vi "set phase sampling info duty cycle.vi"(8 "error in (no error)":errorcluster, 11 "Waveform in":refnum<class "Waveform.lvclass">) -> (0 "error out":errorcluster, 3 "Waveform out":refnum<class "Waveform.lvclass">)   [LabVIEW 2012, in "Waveform.lvclass"]
uses:
  Waveform.lvclass
  Waveform.lvclass/Waveform.ctl
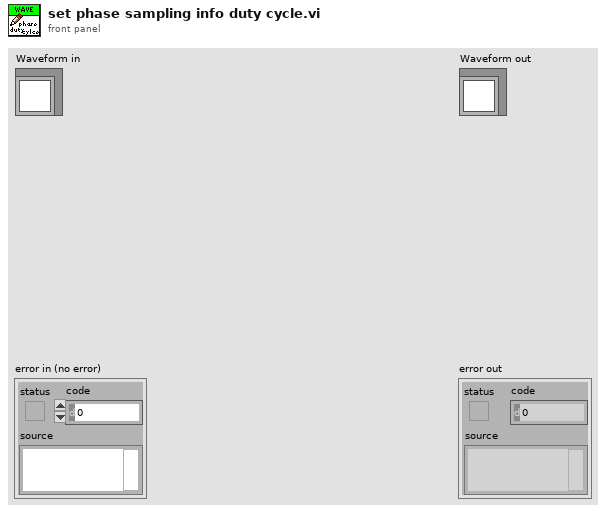
[diagram p1: front panel]
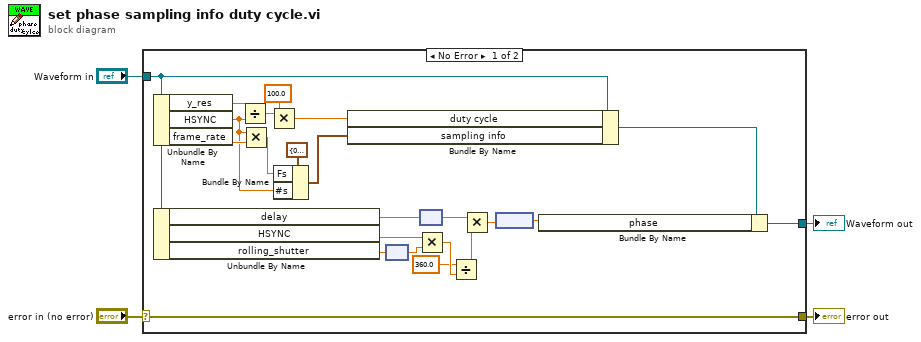
[diagram p0: block diagram]
diagram:
  n1 = case shown="No Error" "error in (no error)" {
    selector: "error in (no error)" -> [w27 w29]
    tunnel: [w27 w29] -> w3
    tunnel: [w11 w28] -> w1
    tunnel: "Waveform in" -> [w17 w28]
    frame No Error {
      n2 = Unbundle By Name(w17) -> ("y_res"=w26:dbl, "HSYNC"=w19:dbl, "frame_rate"=w22:dbl)
      n3 = Unbundle By Name(w17) -> ("delay"=w16:dbl[unit], "HSYNC"=w8:dbl, "rolling_shutter"=w10:dbl[unit])
      n4 = Divide(x=w26, y=w19) -> (x/y=w25:dbl)
      n5 = Multiply(x=w19, y=w22) -> (x*y=w20:dbl)
      n6 = Multiply(x=w25, y=100.0) -> (x*y=w23:dbl)
      n7 = Bundle By Name(cluster=cluster{"Fs":dbl, "#s":dbl} {"Fs"=0.0, "#s"=0.0} ("settings.Pockels Cell.sampling info"), "Fs"=w20, "#s"=w19) -> (w18:cluster{"Fs":dbl, "#s":dbl})
      n8 = Bundle By Name(cluster=w17, "duty cycle"=w23, "sampling info"=w18) -> (w12:refnum<class "Waveform.lvclass">)
      n9 = node(w10) -> (w9:dbl)
      n10 = Multiply(x=w8, y=w9) -> (x*y=w7:dbl)
      n11 = node(w16) -> (w15:dbl)
      n12 = Divide(x=360.0, y=w7) -> (x/y=w5:dbl)
      n13 = Multiply(x=w15, y=w5) -> (x*y=w14:dbl)
      n14 = node(w14) -> (w13:dbl[unit])
      n15 = Bundle By Name(cluster=w12, "phase"=w13) -> (w11:refnum<class "Waveform.lvclass">)
    }
    frame Error {
    }
  }
  "error out" <- w3
  "Waveform out" <- w1
